vi "Read Write.vi"(6 "Read Length":u32, 7 "Write Data":u8[](array[numeric]), 8 "Error In":errorcluster, 9 "Offset":u32 format="%.0x", 10 "Index Group":u32 format="%.0x", 11 "AMS Connection In":T2) -> (0 "Error Out":errorcluster, 1 "Success":bool, 2 "ADS Error":T1 items=["NoError"=0, "InternalError"=1, "NoRTime"=2, "LockedMemoryError"=3, "MailBoxError"=4, "WrongHMsg"=5, "TargetPortNotFound"=6, "TargetMachineNotFound"=7, "UnknownCommandID"=8, "BadTaskID"=9, "NoIO"=10, "UnknownAmsCommand"=11, "Win32Error"=12, "PortNotConnected"=13, "InvalidAmsLength"=14, "InvalidAmsNetID"=15, "AmsSyncAmsError"=22, "AmsSyncNoIndexMap"=23, "InvalidAmsPort"=24, "NoMemory"=25, "TCPSendError"=26, "HostUnreachable"=27, "NoLockedMemory"=1280, "MailboxFull"=1282, "DeviceError"=1792, "DeviceServiceNotSupported"=1793, "DeviceInvalidGroup"=1794, "DeviceInvalidOffset"=1795, "DeviceInvalidAccess"=1796, "DeviceInvalidSize"=1797, "DeviceInvalidData"=1798, "DeviceNotReady"=1799, "DeviceBusy"=1800, "DeviceInvalidContext"=1801, "DeviceNoMemory"=1802, "DeviceInvalidParam"=1803, "DeviceNotFound"=1804, "DeviceSyntaxError"=1805, "DeviceIncompatible"=1806, "DeviceExists"=1807, "DeviceSymbolNotFound"=1808, "DeviceSymbolVersionInvalid"=1809, "DeviceInvalidState"=1810, "DeviceTransModeNotSupported"=1811, "DeviceNotifyHandleInvalid"=1812, "DeviceClientUnknown"=1813, "DeviceNoMoreHandles"=1814, "DeviceInvalidWatchsize"=1815, "DeviceNotInitialized"=1816, "DeviceTimeOut"=1817, "DeviceNoInterface"=1818, "DeviceInvalidInterface"=1819, "DeviceInvalidCLSID"=1820, "DeviceInvalidObjectID"=1821, "ClientError"=1856, "ClientInvalidParameter"=1857, "ClientListEmpty"=1858, "ClientVariableInUse"=1859, "ClientDuplicateInvokeID"=1860, "ClientSyncTimeOut"=1861, "ClientW32OR"=1862, "ClientTimeoutInvalid"=1863, "ClientPortNotOpen"=1864, "ClientNoAmsAddr"=1865, "ClientSyncInternal"=1872, "ClientAddHash"=1873, "ClientRemoveHash"=1874, "ClientNoMoreSymbols"=1875, "ClientSyncResInvalid"=1876, "ClientSyncPortLocked"=1877, "ClientQueueFull"=1878], 3 "Read Data":u8[](array[numeric]) format="%.0x")   [LabVIEW 2020, in "TwinCAT ADS.lvlib"]
uses:
  <userlib>/PMA/TwinCAT ADS.lvlib
  <userlib>/PMA/Low Level/TypeDefs/AMS Connection.ctl
  <userlib>/PMA/Low Level/TypeDefs/AMS.ctl
  <userlib>/PMA/Low Level/TypeDefs/ADS Error.ctl
  <userlib>/PMA/Low Level/TypeDefs/Command Id.ctl
  <userlib>/PMA/Low Level/TypeDefs/State Flag.ctl
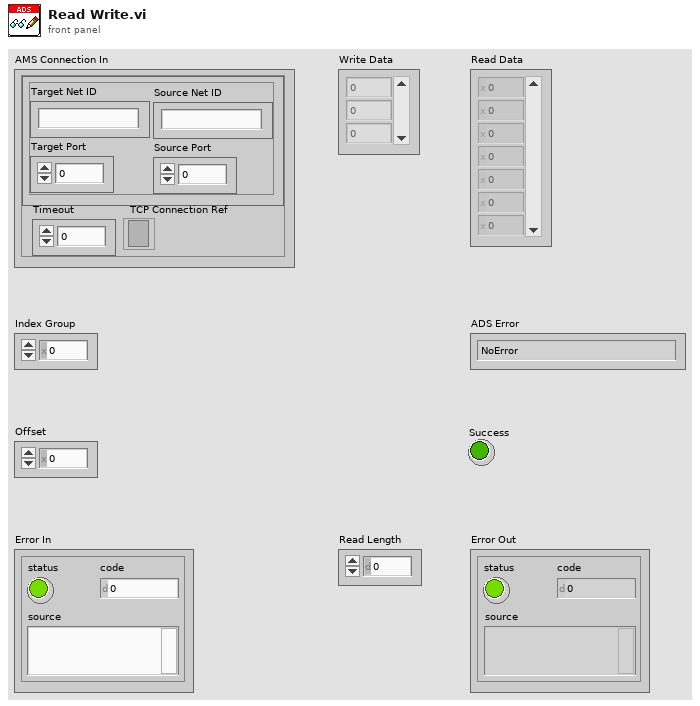
[diagram p1: front panel]
types:
  T1 = typedef "TwinCAT ADS.lvlib/ADS Error.ctl" = i32
  T2 = typedef "TwinCAT ADS.lvlib/AMS Connection.ctl" = cluster{"AMS":T3, "Timeout":i32, "TCP Connection Ref":refnum<k5>}
  T3 = typedef "TwinCAT ADS.lvlib/AMS.ctl" = cluster{"Target Net ID":string, "Target Port":u16, "Source Net ID":string, "Source Port":u16}
  T4 = enum16{"Standard", "Buffered", "CRLF", "Immediate"}
  T5 = typedef "TwinCAT ADS.lvlib/State Flag.ctl" = u16
  T6 = typedef "TwinCAT ADS.lvlib/Command Id.ctl" = enum16{"Invalid", "ADS Read Device Info", "ADS Read", "ADS Write", "ADS Read State", "ADS Write Control", "ADS Add Device Notification", "ADS Delete Device Notification", "ADS Device Notification", "ADS Read Write"}
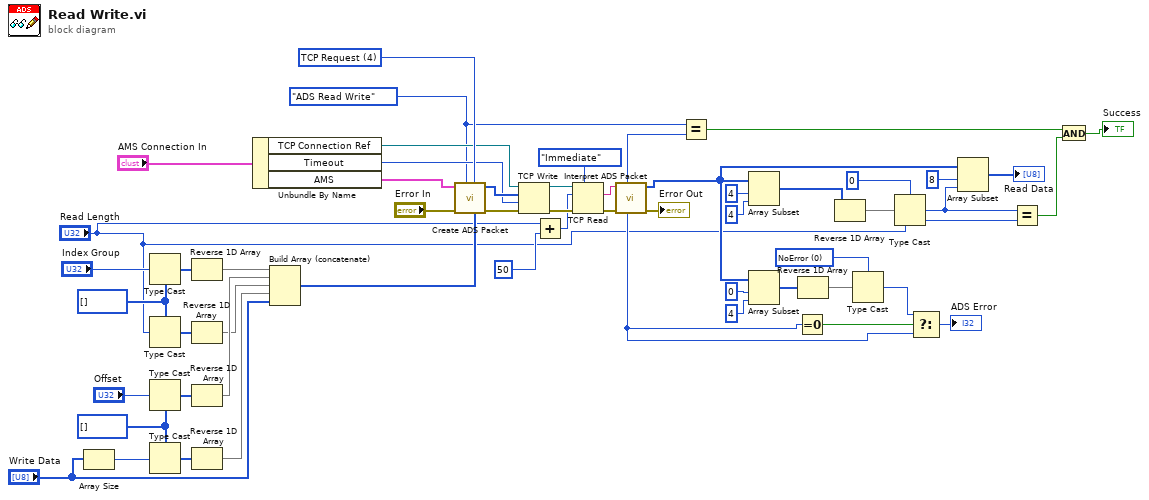
[diagram p0: block diagram]
diagram:
  w10 = u8[] [] ("bytes to read")
  w35 = T1 0 items=["NoError"=0, "InternalError"=1, "NoRTime"=2, "LockedMemoryError"=3, "MailBoxError"=4, "WrongHMsg"=5, "TargetPortNotFound"=6, "TargetMachineNotFound"=7, "UnknownCommandID"=8, "BadTaskID"=9, "NoIO"=10, "UnknownAmsCommand"=11, "Win32Error"=12, "PortNotConnected"=13, "InvalidAmsLength"=14, "InvalidAmsNetID"=15, "AmsSyncAmsError"=22, "AmsSyncNoIndexMap"=23, "InvalidAmsPort"=24, "NoMemory"=25, "TCPSendError"=26, "HostUnreachable"=27, "NoLockedMemory"=1280, "MailboxFull"=1282, "DeviceError"=1792, "DeviceServiceNotSupported"=1793, "DeviceInvalidGroup"=1794, "DeviceInvalidOffset"=1795, "DeviceInvalidAccess"=1796, "DeviceInvalidSize"=1797, "DeviceInvalidData"=1798, "DeviceNotReady"=1799, "DeviceBusy"=1800, "DeviceInvalidContext"=1801, "DeviceNoMemory"=1802, "DeviceInvalidParam"=1803, "DeviceNotFound"=1804, "DeviceSyntaxError"=1805, "DeviceIncompatible"=1806, "DeviceExists"=1807, "DeviceSymbolNotFound"=1808, "DeviceSymbolVersionInvalid"=1809, "DeviceInvalidState"=1810, "DeviceTransModeNotSupported"=1811, "DeviceNotifyHandleInvalid"=1812, "DeviceClientUnknown"=1813, "DeviceNoMoreHandles"=1814, "DeviceInvalidWatchsize"=1815, "DeviceNotInitialized"=1816, "DeviceTimeOut"=1817, "DeviceNoInterface"=1818, "DeviceInvalidInterface"=1819, "DeviceInvalidCLSID"=1820, "DeviceInvalidObjectID"=1821, "ClientError"=1856, "ClientInvalidParameter"=1857, "ClientListEmpty"=1858, "ClientVariableInUse"=1859, "ClientDuplicateInvokeID"=1860, "ClientSyncTimeOut"=1861, "ClientW32OR"=1862, "ClientTimeoutInvalid"=1863, "ClientPortNotOpen"=1864, "ClientNoAmsAddr"=1865, "ClientSyncInternal"=1872, "ClientAddHash"=1873, "ClientRemoveHash"=1874, "ClientNoMoreSymbols"=1875, "ClientSyncResInvalid"=1876, "ClientSyncPortLocked"=1877, "ClientQueueFull"=1878] ("Enum")
  w11 = u8[] [] ("bytes to read")
  w55 = T5 4 items=["TCP Request"=4, "TCP Response"=5, "UDP Request"=68, "UDP Respone"=69] ("State Flag")
  w8 = Command_Id."ADS Read Write" ("Command ID")
  n1 = Array Size(array="Write Data") -> (size(s)=w12:i32)
  n2 = Type Cast(type=w11, x="Index Group") -> (*(type *) &x=w42:u8[])
  n3 = Type Cast(type=w11, x="Read Length") -> (*(type *) &x=w40:u8[])
  n4 = Type Cast(type=w10, x="Offset") -> (*(type *) &x=w41:u8[])
  n5 = Type Cast(type=w10, x=w12) -> (*(type *) &x=w18:u8[])
  n6 = Reverse 1D Array(array=w42) -> (reversed array=w26:u8[])
  n7 = Reverse 1D Array(array=w40) -> (reversed array=w24:u8[])
  n8 = Reverse 1D Array(array=w41) -> (reversed array=w25:u8[])
  n9 = Reverse 1D Array(array=w18) -> (reversed array=w17:u8[])
  n10 = Unbundle By Name("AMS Connection In") -> ("TCP Connection Ref"=w14:refnum<k5>, "Timeout"=w15:i32, "AMS"=w16:T3)
  n11 = Build Array (concatenate)(w26, w25, w24, w17, "Write Data") -> (w39:u8[])
  n12 = call <userlib>:"Create ADS Packet.vi"("Data"=w39, "State Flag"=w55, "Command ID"=w8, "Error In"="Error In", "AMS"=w16) -> ("Error Out"=w52:errorcluster, "ADS Packet"=w54:u8[])  [unwired: 5 in]
  n13 = TCP Write(connection ID=w14, data in=w54, error in (no error)=w52, 9:w15) -> (connection ID out=w53:refnum<k5>, error out=w51:errorcluster)  [unwired: 1 out]
  n14 = Add(x="Read Length", y=u32 50 ("bytes to read")) -> (x+y=w27:u32)
  n15 = TCP Read(connection ID=w53, bytes to read=w27, error in (no error)=w51, 7:T4."Immediate" ("mode (standard)")) -> (data out=w46:string, error out=w47:errorcluster)  [unwired: 1 in, 1 out]
  n16 = call <userlib>:"Interpret ADS Packet.vi"("Error In"=w47, "ADS Packet"=w46) -> ("Error Out"=→"Error Out":errorcluster, "Data"=w30:u8[], "ADS Error"=w20:T1, "Command ID"=w7:T6)  [unwired: 3 in, 3 out]
  n17 = Equal?(x=w8, y=w7) -> (x = y?=w3:bool)
  n18 = Array Subset(array=w30, index=4, length=4) -> (w32:u8[])
  n19 = Array Subset(array=w30, index=0, length=4) -> (w36:u8[])
  n20 = Equal To 0?(x=w20) -> (x = 0?=w22:bool)
  n21 = Reverse 1D Array(array=w36) -> (reversed array=w23:u8[])
  n22 = Reverse 1D Array(array=w32) -> (reversed array=w1:u8[])
  n23 = Type Cast(type=w35, x=w23) -> (*(type *) &x=w21:T1)
  n24 = Type Cast(type=u32 0 ("bytes to read"), x=w1) -> (*(type *) &x=w5:u32)
  n25 = Select(t=w21, s=w22, f=w20) -> (s? t:f=→"ADS Error":T1)
  n26 = Array Subset(array=w30, index=8, length=w5) -> (→"Read Data":u8[])
  n27 = Equal?(x=w5, y="Read Length") -> (x = y?=w2:bool)
  n28 = And(x=w3, y=w2) -> (x .and. y?=→"Success":bool)
